vi "niRFUtil MT UTIL Validate Samples Per Symbol.vi"(11 "Samples Per Symbol":i32=16) -> (0 "error out":errorcluster, 1 "error?":bool)   [LabVIEW 2015, in "niRFUtil.lvlib"]
doc: "Verifies that the provided System Parameters are valid based on:\n1. Samples/Symbol must be greater than zero.\n2. Samples/Symbol must be even.\n3. Symbol Rate must be greater than zero."
uses:
  niRFUtil.lvlib
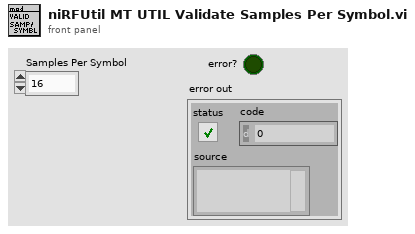
[diagram p1: front panel]
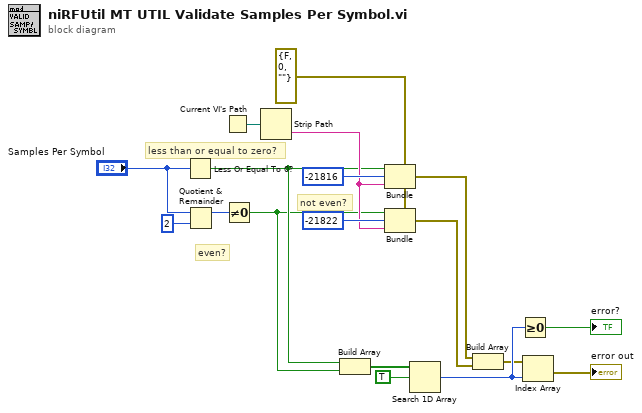
[diagram p0: block diagram]
diagram:
  w1 = errorcluster {"status"=FALSE, "code"=0, "source"=""} ("error out")
  # "even?"
  # "less than or equal to zero?"
  # "not even?"
  n1 = Less Or Equal To 0?(x="Samples Per Symbol") -> (x <= 0?=w5:bool)
  n2 = Quotient & Remainder(x="Samples Per Symbol", y=2) -> (x-y*floor(x/y)=w10:i32)  [unwired: 1 out]
  n3 = Current VI's Path() -> (path=w17:path)
  n4 = Not Equal To 0?(x=w10) -> (x != 0?=w4:bool)
  n5 = Strip Path(path=w17) -> (name=w8:string)  [unwired: 1 out]
  n6 = Build Array(w5, w4) -> (w14:bool[])
  n7 = Bundle(cluster=w1, "status"=w5, "code"=-21816, "source"=w8) -> (w7:errorcluster)
  n8 = Bundle(cluster=w1, "status"=w4, "code"=-21822, "source"=w8) -> (w6:errorcluster)
  n9 = Search 1D Array(1D array=w14, element=TRUE) -> (index of element=w15:i32)  [unwired: 1 out]
  n10 = Build Array(w7, w6) -> (w12:errorcluster[])
  n11 = Greater Or Equal To 0?(x=w15) -> (x >= 0?=→"error?":bool)
  n12 = Index Array(array=w12, index=w15) -> (element=→"error out":errorcluster)
